vi "Read from TDMS File.vi"(7 "Track Name":string, 8 "Error In":errorcluster, 9 "Number of Elements":i64, 10 "Read Position":i64, 11 "TDMS Reference In":refnum<k34>) -> (0 "Error Out":errorcluster, 2 "Audio Out":T1, 3 "TDMS Reference Out":refnum<k34>)   [LabVIEW 2014]
doc: "This function will read back track data from the specified Track. You can specify the position in the file to start reading from and the number of elements to be read."
uses:
  Controls/Audio In.ctl
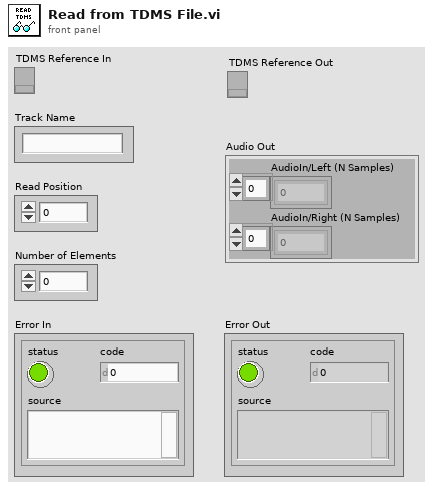
[diagram p1: front panel]
types:
  T1 = typedef "Audio In.ctl" = cluster{"AudioIn/Left (N Samples)":i16[], "AudioIn/Right (N Samples)":i16[]}
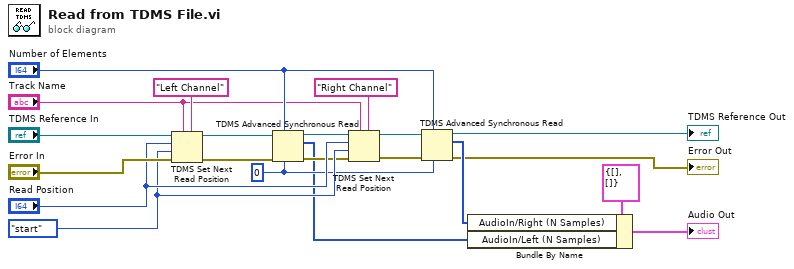
[diagram p0: block diagram]
diagram:
  w10 = i16 0 ("data type")
  w15 = enum16{"start", "end"}."start" ("from (0: start)")
  n1 = TDMS Set Next Read Position(5:"Left Channel" ("channel name in"), 7:"Track Name", 8:"Error In", 9:w15, 10:"Read Position", 11:"TDMS Reference In") -> (0:w18:errorcluster, 3:w17:refnum<k34>)
  n2 = TDMS Advanced Synchronous Read(6:w10, 7:"Number of Elements", 8:w18, 11:w17) -> (0:w14:errorcluster, 2:w4:i16[], 3:w13:refnum<k34>)  [unwired: 1 out]
  n3 = TDMS Set Next Read Position(5:"Right Channel" ("channel name in"), 7:"Track Name", 8:w14, 9:w15, 10:"Read Position", 11:w13) -> (0:w11:errorcluster, 3:w12:refnum<k34>)
  n4 = TDMS Advanced Synchronous Read(6:w10, 7:"Number of Elements", 8:w11, 11:w12) -> (0:→"Error Out":errorcluster, 2:w5:i16[], 3:→"TDMS Reference Out":refnum<k34>)  [unwired: 1 out]
  n5 = Bundle By Name(cluster=T1 {"AudioIn/Left (N Samples)"=[], "AudioIn/Right (N Samples)"=[]} ("Audio In"), "AudioIn/Right (N Samples)"=w5, "AudioIn/Left (N Samples)"=w4) -> (→"Audio Out":T1)
